vi "Replase ALR_ON_OFFs.vi"(8 "error in (no error)":errorcluster, 9 "Data":bool[](array[boolean]), 10 "Index":i32[](array[numeric]), 11 "ALR_ON_OFF":refnum<data-value>) -> (0 "error out":errorcluster, 3 "ALR_ON_OFF out":refnum<data-value>)   [LabVIEW 2019, in "Alarms.lvlib"]
uses:
  Alarms.lvlib
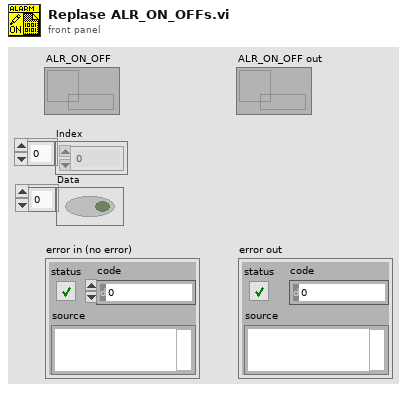
[diagram p1: front panel]
types:
  T1 = cluster{"ALR_ON":bool[], "ALR_OFF":bool[], "ALR_reset":bool[], "ALR_check":bool[], "ALR_block":bool[], "ALR_Ack":bool[]}
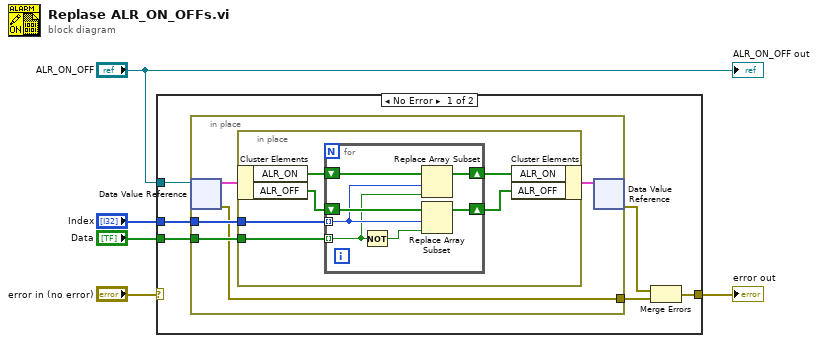
[diagram p0: block diagram]
diagram:
  n1 = case shown="No Error" "error in (no error)" {
    selector: "error in (no error)" -> [_ w30]
    tunnel: "Index" -> [w11 _]
    tunnel: [w6 w30] -> w4
    tunnel: "ALR_ON_OFF" -> [w10 _]
    tunnel: "Data" -> [w9 _]
    frame No Error {
      n2 = in-place {
        in-place-border: w11 -> [w15]
        in-place-border: w9 -> [w14]
        in-place-border: [w12] -> w7
        n3 = in-place-dvr #1(w10) -> (w16:T1, w12:errorcluster)
        n4 = in-place {
          in-place-border: w15 -> [w21]
          in-place-border: w14 -> [w19]
          n5 = in-place-cluster #2(w16) -> ("ALR_ON"=w22:bool[], "ALR_OFF"=w20:bool[])
          n6 = for {
            tunnel: w21 -> [w27] mode=indexing
            tunnel: w19 -> [w26] mode=indexing
            shift-right: [w25] -> w18
            shift-left: w22 -> [w29]
            shift-right: [w24] -> w17
            shift-left: w20 -> [w28]
            n7 = Not(x=w26) -> (.not. x?=w23:bool)
            n8 = Replace Array Subset(array=w29, new element=w26, index=w27) -> (w25:bool[])
            n9 = Replace Array Subset(array=w28, new element=w23, index=w27) -> (w24:bool[])
          }
          n10 = in-place-cluster #2("ALR_ON"=w18, "ALR_OFF"=w17) -> (w13:T1)
        }
        n11 = in-place-dvr #1(w13) -> (w8:errorcluster)  [unwired: 1 out]
      }
      n12 = Merge Errors(w8, w7) -> (w6:errorcluster)
    }
    frame Error {
    }
  }
  "error out" <- w4
  "ALR_ON_OFF out" <- "ALR_ON_OFF"
